vi "DirectFFTtoSound.vi"() -> ()   [LabVIEW 2014]
uses:
  <vilib>/Analysis/2dsp.llb/Inverse Real FFT.vi
  <vilib>/Analysis/NI_AALPro.lvlib
panel:
  out "Waveform Graph 3":waveform(dbl)(graph)
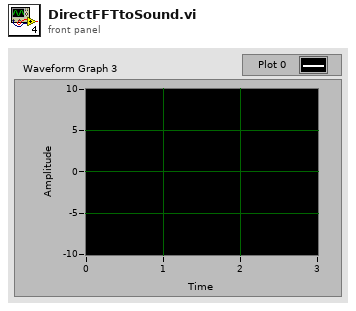
[diagram p1: front panel]
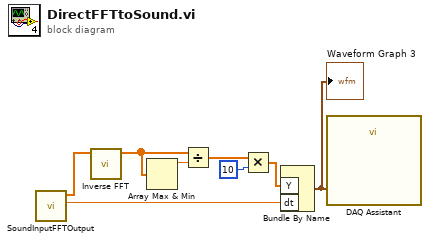
[diagram p0: block diagram]
diagram:
  n1 = call "SoundInputFFTOutput.vi"() -> ("dt"=w1:dbl, "FFT {X}"=w6:cdb[])  [unwired: 10 in]
  n2 = call-poly <vilib>:"Inverse FFT.vi"("FFT {X}"=w6) -> ("X"=w4:dbl[])  [unwired: 9 in, 1 out]
  n3 = Array Max & Min(array=w4) -> (max value=w5:dbl)  [unwired: 3 out]
  n4 = Divide(x=w4, y=w5) -> (x/y=w8:dbl[])
  n5 = Multiply(x=w8, y=10) -> (x*y=w3:dbl[])
  n6 = Bundle By Name("Y"=w3, "dt"=w1) -> (w2:waveform(dbl))  [unwired: 1 in]
  "Waveform Graph 3" <- w2
  n7 = call "DAQ Assistant"("data"=w2) -> ()  [unwired: 17 in, 2 out]
